vi "试剂余量后台任务.vi"   [LabVIEW 2016, in "斯坦道CODMn新电路板.lvlib"]
uses:
  <vilib>/ptbypt/NI_PtbyPt.lvlib
types:
  T1 = cluster{"V1":sgl, "V2":sgl, "V3":sgl, "V4":sgl, "V5":sgl, "V6":sgl, "V7":sgl, "V8":sgl, "V9":sgl, "V10":sgl, "V11":sgl, "V12":sgl, "V9-1":sgl, "V9-2":sgl}
  T2 = cluster{"时间标识":timestamp, "设备":string, "日志信息":string, "备注":string}
  T3 = cluster{"系统时间":timestamp, "工作状态":u16, "测量模式":enum16{"待机", "连续模式", "周期模式", "定点模式", "受控模式", "手动模式"}, "告警代码":u16, "故障代码":u16, "日志代码":u16, "软件版本":u16, "A":sgl, "B":sgl, "K":sgl, "当前滴定数":sgl, "T":sgl, "H":sgl, "id":u16, "flowid":u16, "量程":u16, "加热实时温度":sgl, "当前ORP值":sgl, "运行时间":sgl, "当前步骤剩余时间":sgl, "结束滴定数":sgl, "注射泵保温温度":sgl, "匹配滴定数X0":u16, "X^2":sgl, "X":sgl, "B 2":sgl}
  T4 = cluster{"V1":bool, "V2":bool, "V3":bool, "V4":bool, "V5":bool, "V6":bool, "V7":bool, "V8":bool, "V9":bool, "V10":bool, "V11":bool, "V12":bool, "V9-1":bool, "V9-2":bool}
  T5 = cluster{"参数":string, "报警内容":string, "报警分析":string}
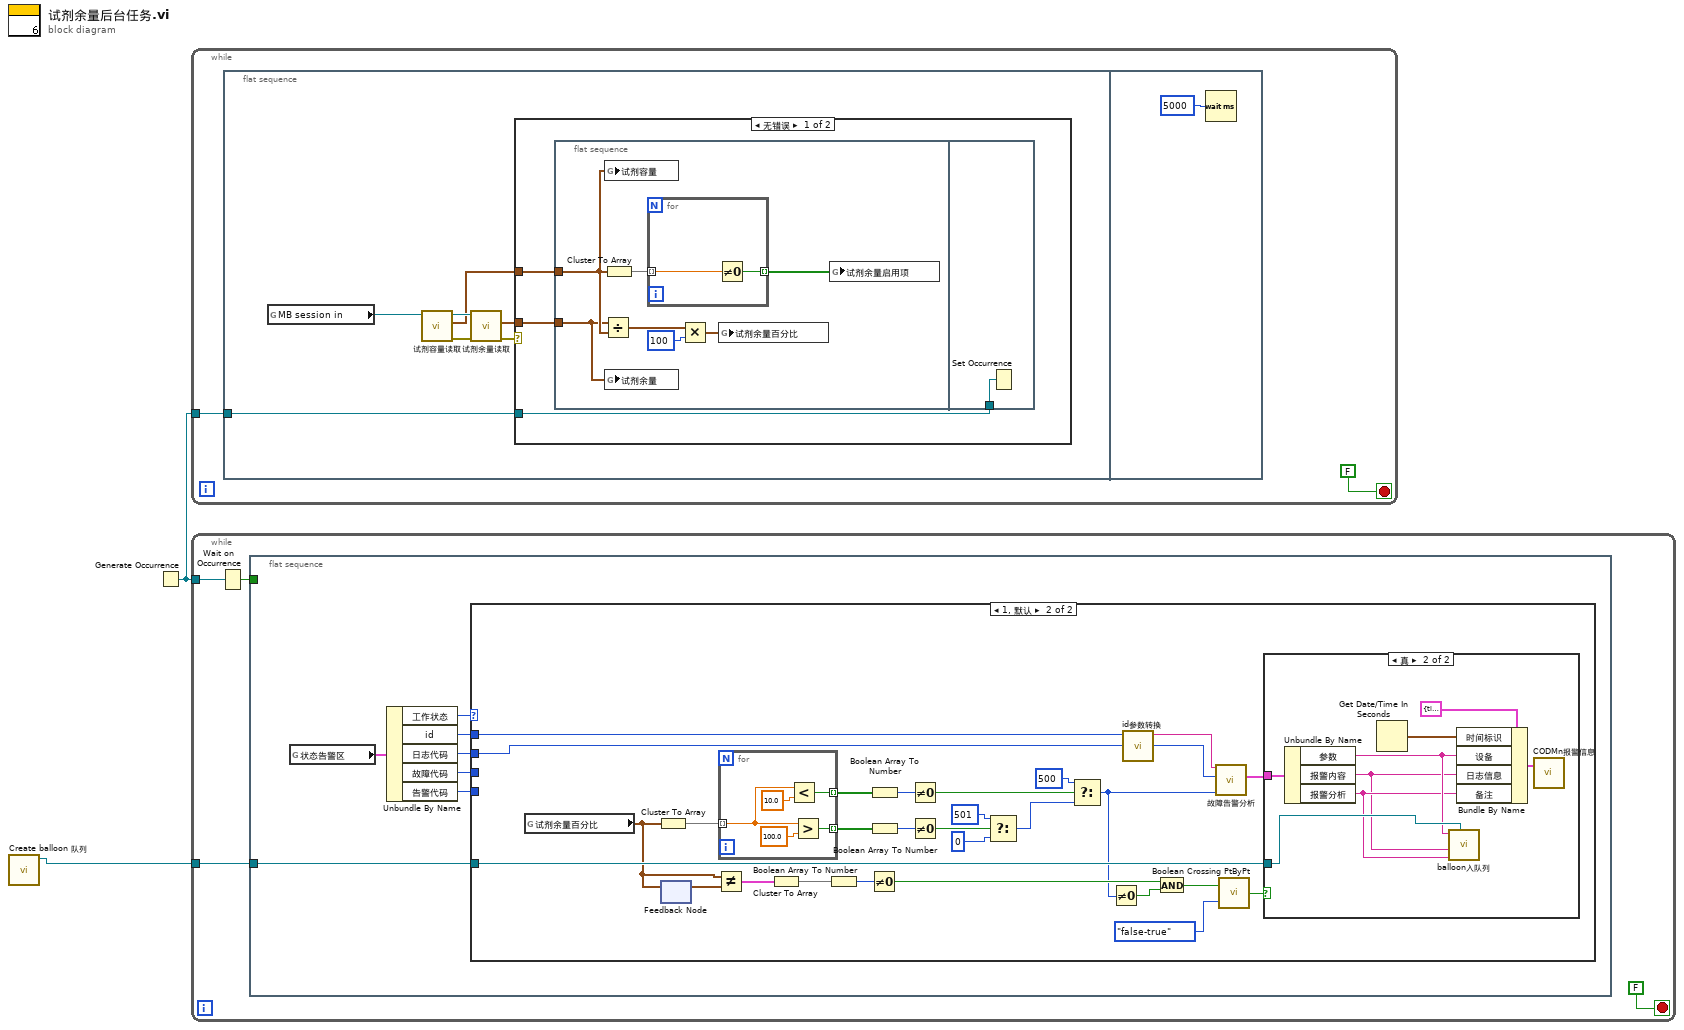
[diagram p0: block diagram]
diagram:
  n1 = call "Create balloon 队列.vi"() -> ("队列输出"=w1:refnum<queue>)  [unwired: 11 in]
  n2 = Generate Occurrence() -> (w2:refnum<k4>)
  n3 = while {
    tunnel: w2 -> [w3]
    stop <- FALSE stop-if-true
    n4 = flat-sequence {
      tunnel: w3 -> [w5]
      frame #0 {
        n5 = global read "VARCODMn全局变量.vi" "MB session in"() -> (w9:refnum<class "MB_Master.lvclass">)
        n6 = call "试剂容量读取.vi"("MB session in"=w9) -> ("error out"=w11:errorcluster, "试剂容量"=w8:T1, "MB session out"=w10:refnum<class "MB_Master.lvclass">)  [unwired: 8 in]
        n7 = call "试剂余量读取.vi"("Error in"=w11, "MB session in"=w10) -> ("error out"=w6:errorcluster, "试剂余量"=w7:T1)  [unwired: 7 in, 1 out]
        n8 = case shown="无错误" w6 {
          tunnel: w8 -> [w14 _]
          tunnel: w7 -> [w13 _]
          tunnel: w5 -> [w12 _]
          frame No Error {
            n9 = flat-sequence {
              tunnel: w14 -> [w19]
              tunnel: w13 -> [w18]
              tunnel: w12 -> [w24]
              frame #0 {
                n10 = Divide(x=w18, y=w19) -> (x/y=w21:T1)
                n11 = Cluster To Array(cluster=w19) -> (array=w16:sgl[])
                n12 = global write "VARCODMn全局变量.vi" "试剂容量"(w19) -> ()
                n13 = global write "VARCODMn全局变量.vi" "试剂余量"(w18) -> ()
                n14 = for {
                  tunnel: w16 -> [w23] mode=indexing
                  tunnel: [w22] -> w15 mode=indexing
                  n15 = Not Equal To 0?(x=w23) -> (x != 0?=w22:bool)
                }
                n16 = Multiply(x=w21, y=100) -> (x*y=w17:T1)
                n17 = global write "VARCODMn全局变量.vi" "试剂余量百分比"(w17) -> ()
                n18 = global write "VARCODMn全局变量.vi" "试剂余量启用项"(w15) -> ()
              }
              frame #1 {
                n19 = Set Occurrence(w24) -> ()
              }
            }
          }
          frame Error {
          }
        }
      }
      frame #1 {
        n20 = Wait (ms)(milliseconds to wait=u32 5000 ("等待时间（毫秒）")) -> ()  [unwired: 1 out]
      }
    }
  }
  n21 = while {
    tunnel: w1 -> [w28]
    tunnel: w2 -> [w27]
    stop <- FALSE stop-if-true
    n22 = Wait on Occurrence(2:w27) -> (0:w26:bool)  [unwired: 2 in]
    n23 = flat-sequence {
      tunnel: w28 -> [w34]
      tunnel: w26 -> [_]
      frame #0 {
        n24 = global read "VARCODMn全局变量.vi" "状态告警区"() -> (w30:T3)
        n25 = Unbundle By Name(w30) -> ("工作状态"=w31:u16, "id"=w36:u16, "日志代码"=w35:u16, "故障代码"=w33:u16, "告警代码"=w32:u16)
        n26 = case shown="1, 默认" w31 {
          tunnel: w36 -> [_ w41]
          tunnel: w35 -> [_ w37]
          tunnel: w34 -> [_ w63]
          tunnel: w33 -> [_ _]
          tunnel: w32 -> [_ _]
          frame 0 {
          }
          frame 1, Default {
            n27 = global read "VARCODMn全局变量.vi" "试剂余量百分比"() -> (w49:T1)
            n28 = Cluster To Array(cluster=w49) -> (array=w58:sgl[])
            n29 = feedback-in #1(w49) -> ()
            n30 = feedback #1() -> (w50:T1)  [unwired: 1 in]
            n31 = Not Equal?(x=w49, y=w50) -> (x != y?=w48:T4)
            n32 = for {
              tunnel: w58 -> [w66] mode=indexing
              tunnel: [w67] -> w60 mode=indexing
              tunnel: [w64] -> w59 mode=indexing
              n33 = Less?(x=w66, y=sgl 10.0) -> (x < y?=w67:bool)
              n34 = Greater?(x=w66, y=sgl 100.0) -> (0:w64:bool)
            }
            n35 = Cluster To Array(cluster=w48) -> (array=w47:bool[])
            n36 = Boolean Array To Number(Boolean array=w47) -> (number=w46:u32)
            n37 = Not Equal To 0?(x=w46) -> (x != 0?=w44:bool)
            n38 = Boolean Array To Number(Boolean array=w60) -> (number=w62:u32)
            n39 = Boolean Array To Number(Boolean array=w59) -> (number=w61:u32)
            n40 = Not Equal To 0?(x=w62) -> (x != 0?=w57:bool)
            n41 = Not Equal To 0?(x=w61) -> (x != 0?=w55:bool)
            n42 = Select(t=501, s=w55, f=0) -> (s? t:f=w52:i32)
            n43 = Select(t=500, s=w57, f=w52) -> (s? t:f=w39:i32)
            n44 = Not Equal To 0?(x=w39) -> (x != 0?=w51:bool)
            n45 = call "id参数转换.vi"("id"=w41) -> ("table输出"=w40:string)  [unwired: 10 in]
            n46 = And(x=w44, y=w51) -> (x .and. y?=w45:bool)
            n47 = call "故障告警分析.vi"("告警代码"=w39, "运行步序"=w37, "参数"=w40) -> ("报警内容"=w38:T5)  [unwired: 7 in, 1 out]
            n48 = call <vilib>:"Boolean Crossing PtByPt.vi"("direction"=enum16{"either", "false-true", "true-false"}."false-true", "input"=w45) -> ("crossing"=w43:bool)  [unwired: 1 in]
            n49 = case shown="真" w43 {
              tunnel: w38 -> [_ w76]
              tunnel: w63 -> [_ w73]
              frame False {
              }
              frame True {
                n50 = Unbundle By Name(w76) -> ("参数"=w72:string, "报警内容"=w69:string, "报警分析"=w70:string)
                n51 = Get Date/Time In Seconds() -> (seconds since 1Jan1904=w75:timestamp)
                n52 = call "balloon入队列.vi"("队列"=w73, "故障详情"=w70, "告警信息"=w69, "参数名称"=w72) -> ()  [unwired: 7 in, 1 out]
                n53 = Bundle By Name(cluster=T2 {"时间标识"=timestamp(0 s since 1904-01-01), "设备"="", "日志信息"="", "备注"=""} ("data in"), "时间标识"=w75, "设备"=w72, "日志信息"=w69, "备注"=w70) -> (w71:T2)
                n54 = call "CODMn报警信息.vi"("data in"=w71) -> ()  [unwired: 10 in, 1 out]
              }
            }
          }
        }
      }
    }
  }
